vi "FlatToRichpumploop_Valves.vi"(5 "OutputClusterType":T1, 11 "InputCluster":T2) -> (3 "OutputCluster":T1)   [LabVIEW 2024, in "pumploop_client.lvlib"]
uses:
  pumploop_client.lvlib
  pumploop_Valves_Flat.ctl
  pumploop_Valves.ctl
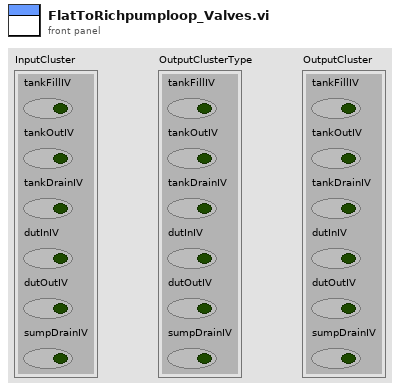
[diagram p1: front panel]
types:
  T1 = typedef "pumploop_client.lvlib/pumploop_Valves.ctl" = cluster{"tankFillIV":bool, "tankOutIV":bool, "tankDrainIV":bool, "dutInIV":bool, "dutOutIV":bool, "sumpDrainIV":bool}
  T2 = typedef "pumploop_client.lvlib/pumploop_Valves_Flat.ctl" = cluster{"tankFillIV":bool, "tankOutIV":bool, "tankDrainIV":bool, "dutInIV":bool, "dutOutIV":bool, "sumpDrainIV":bool}
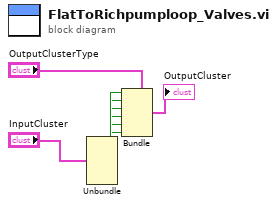
[diagram p0: block diagram]
diagram:
  n1 = Unbundle "Unbundle"("InputCluster") -> ("tankFillIV"=w6:bool, "tankOutIV"=w5:bool, "tankDrainIV"=w4:bool, "dutInIV"=w3:bool, "dutOutIV"=w2:bool, "sumpDrainIV"=w1:bool)
  n2 = Bundle "Bundle"(cluster="OutputClusterType", "tankFillIV"=w6, "tankOutIV"=w5, "tankDrainIV"=w4, "dutInIV"=w3, "dutOutIV"=w2, "sumpDrainIV"=w1) -> (→"OutputCluster":T1)
